vi "HFRR ADV v020 new software.vi"() -> ()   [LabVIEW 2025] (continued)
                  n3417 = local write "S 59"(w4556) -> ()
                }
                frame 59 {
                  n3418 = local write "S 60"(w4557) -> ()
                }
                frame 60 {
                  n3419 = local write "S 62"(w4558) -> ()
                }
                frame 61 {
                  n3420 = local write "S 63"(w4559) -> ()
                }
                frame 62 {
                  n3421 = local write "S 64"(w4560) -> ()
                }
                frame 63 {
                  n3422 = local write "S 65"(w4561) -> ()
                }
                frame 64 {
                  n3423 = local write "S 66"(w4562) -> ()
                }
                frame 65 {
                  n3424 = local write "S 67"(w4563) -> ()
                }
                frame 66 {
                  n3425 = local write "S 68"(w4564) -> ()
                }
                frame 67 {
                  n3426 = local write "S 69"(w4565) -> ()
                }
                frame 68 {
                  n3427 = local write "S 70"(w4566) -> ()
                }
                frame 69 {
                  n3428 = local write "S 71"(w4567) -> ()
                }
                frame 70 {
                  n3429 = local write "S 72"(w4568) -> ()
                }
                frame 71 {
                  n3430 = local write "S 73"(w4569) -> ()
                }
                frame 72 {
                  n3431 = local write "S 74"(w4570) -> ()
                }
                frame 73 {
                  n3432 = local write "S 75"(w4571) -> ()
                }
                frame 74 {
                  n3433 = local write "S 76"(w4572) -> ()
                }
                frame 75 {
                  n3434 = local write "S 77"(w4573) -> ()
                }
                frame 76 {
                  n3435 = local write "S 78"(w4574) -> ()
                }
                frame 77 {
                  n3436 = local write "S 79"(w4575) -> ()
                }
                frame 79 {
                  n3437 = property on="Sample Temperature ( °C )" class="XYGraph (strict)"("Y Scale.Name Label.Text"=w4576) -> ()  [unwired: 2 in, 2 out]
                }
                frame 80 {
                  n3438 = local write "S 81"(w4577) -> ()
                  n3439 = property on="Humidity ( %RH )" class="XYGraph (strict)"("Y Scale.Name Label.Text"=w4577) -> ()  [unwired: 2 in, 2 out]
                }
                frame 78 {
                  n3440 = property on="Air Temperature  ( °C )" class="XYGraph (strict)"("X Scale.Name Label.Text"=w4578) -> ()  [unwired: 2 in, 2 out]
                  n3441 = property on="Humidity ( %RH )" class="XYGraph (strict)"("X Scale.Name Label.Text"=w4578) -> ()  [unwired: 2 in, 2 out]
                  n3442 = property on="Sample Temperature ( °C )" class="XYGraph (strict)"("X Scale.Name Label.Text"=w4578) -> ()  [unwired: 2 in, 2 out]
                  n3443 = property on="Coefficient Of Friction" class="XYGraph (strict)"("X Scale.Name Label.Text"=w4578) -> ()  [unwired: 2 in, 2 out]
                }
                frame 81 {
                  n3444 = property on="Air Temperature  ( °C )" class="XYGraph (strict)"("Y Scale.Name Label.Text"=w4579) -> ()  [unwired: 2 in, 2 out]
                }
                frame 82 {
                  n3445 = local write "S 84"(w4580) -> ()
                }
                frame 83 {
                  n3446 = local write "S 85"(w4581) -> ()
                }
                frame 84 {
                  n3447 = local write "S 86"(w4582) -> ()
                }
                frame 85 {
                  n3448 = local write "S 87"(w4583) -> ()
                }
                frame 86 {
                  n3449 = local write "S 88"(w4584) -> ()
                }
                frame 87 {
                }
                frame 88 {
                  n3450 = local write "S 90"(w4586) -> ()
                }
                frame 89 {
                  n3451 = local write "S 91"(w4587) -> ()
                }
                frame 90 {
                  n3452 = local write "S 92"(w4588) -> ()
                }
                frame 91 {
                  n3453 = local write "S 93"(w4589) -> ()
                }
                frame 92 {
                  n3454 = local write "S 94"(w4590) -> ()
                }
                frame 93 {
                  n3455 = local write "S 95"(w4591) -> ()
                }
                frame 94 {
                  n3456 = local write "S 96"(w4592) -> ()
                }
                frame 95 {
                  n3457 = local write "S 97"(w4593) -> ()
                }
                frame 96 {
                  n3458 = local write "S 98"(w4594) -> ()
                }
                frame 97 {
                  n3459 = local write "S 99"(w4595) -> ()
                }
                frame 98 {
                  n3460 = local write "S 100"(w4596) -> ()
                }
                frame 99 {
                  n3461 = local write "S 101"(w4597) -> ()
                }
                frame 100 {
                  n3462 = local write "S 102"(w4598) -> ()
                }
                frame 101 {
                  n3463 = local write "S 103"(w4599) -> ()
                }
                frame 102 {
                  n3464 = local write "S 104"(w4600) -> ()
                }
                frame 103 {
                  n3465 = local write "S 105"(w4601) -> ()
                }
                frame 104 {
                  n3466 = local write "S 106"(w4602) -> ()
                }
                frame 105 {
                }
                frame 106 {
                  n3467 = property on="OK Button 17" class="Bool (strict)"("Boolean Text.Text"=w4603) -> ()  [unwired: 2 in, 2 out]
                }
                frame 107 {
                  n3468 = property on="OK Button 16" class="Bool (strict)"("Boolean Text.Text"=w4604) -> ()  [unwired: 2 in, 2 out]
                }
                frame 108 {
                  n3469 = property on="TITTLE" class="Str"("Caption.Text"=w4605) -> ()  [unwired: 2 in, 2 out]
                }
                frame 109 {
                  "String 30" <- w4606
                }
                frame 110 {
                  n3470 = property on="Test Date" class="Str"("Caption.Text"=w4607) -> ()  [unwired: 2 in, 2 out]
                  "String 31" <- w4607
                }
                frame 111 {
                  n3471 = property on="Sample ID" class="Str"("Caption.Text"=w4608) -> ()  [unwired: 2 in, 2 out]
                  "String 32" <- w4608
                }
                frame 112 {
                  n3472 = property on="Tested by" class="Str"("Caption.Text"=w4609) -> ()  [unwired: 2 in, 2 out]
                  "String 33" <- w4609
                }
                frame 113 {
                  n3473 = property on="System Configured Printers 2" class="Arr (strict)"("Caption.Text"=w4610) -> ()  [unwired: 2 in, 2 out]
                }
                frame 114 {
                  n3474 = property on="Selected Printer" class="Str"("Caption.Text"=w4611) -> ()  [unwired: 2 in, 2 out]
                }
                frame 115 {
                  n3475 = property on="Select Printer 3" class="DigNum (strict)"("Caption.Text"=w4612) -> ()  [unwired: 2 in, 2 out]
                }
                frame 116 {
                  n3476 = property on="Print" class="Bool (strict)"("Boolean Text.Text"=w4613) -> ()  [unwired: 2 in, 2 out]
                }
                frame 117 {
                  "String 41" <- w4614
                }
                frame 118 {
                  n3477 = property on="tested by" class="Str"("Caption.Text"=w4615) -> ()  [unwired: 2 in, 2 out]
                }
                frame 119 {
                }
                frame 120 {
                  n3478 = property on="Export" class="Bool (strict)"("Boolean Text.Text"=w4616) -> ()  [unwired: 2 in, 2 out]
                }
                frame 121 {
                  n3479 = property on="TEMP INTERCEPT:" class="DigNum (strict)"("Caption.Text"=w4617) -> ()  [unwired: 2 in, 2 out]
                }
                frame 122 {
                  n3480 = property on="AIR TEMP INTERCEPT:" class="DigNum (strict)"("Caption.Text"=w4618) -> ()  [unwired: 2 in, 2 out]
                }
                frame 123 {
                  n3481 = property on="Select File Type" class="Enum (strict)"("Caption.Text"=w4619) -> ()  [unwired: 2 in, 2 out]
                }
                frame 124 {
                  n3482 = property on="s.NO" class="Str"("Caption.Text"=w4620) -> ()  [unwired: 2 in, 2 out]
                  "String 45" <- w4620
                }
                frame 125 {
                  n3483 = property on="trip1 8" class="Bool (strict)"("Boolean Text.Text"=w4621) -> ()  [unwired: 2 in, 2 out]
                }
                frame 126, Default {
                }
              }
            }
          }
          frame #1 {
            w4629 = TRUE ("Visible")
            n3484 = local read "S 91"() -> (w4646:string)
            n3485 = local read "S 90"() -> (w4645:string)
            n3486 = local read "S 88"() -> (w4644:string)
            n3487 = property on="File Path" class="Path"("Caption.Text"=w4645) -> ()  [unwired: 2 in, 2 out]
            n3488 = property on="SrvM CP" class="Bool (strict)"("Boolean Text.Text"=w4644) -> ()  [unwired: 2 in, 2 out]
            n3489 = local read "S 71"() -> (w4639:string)
            n3490 = local read "S 86"() -> (w4641:string)
            n3491 = local read "S 85"() -> (w4642:string)
            n3492 = local read "S 87"() -> (w4640:string)
            n3493 = local read "S 84"() -> (w4643:string)
            n3494 = local read "S 103"() -> (w4628:string)
            n3495 = local read "S 104"() -> (w4627:string)
            n3496 = property on="ENTER THE NEW PASSWORD" class="Str"("Caption.Text"=w4640) -> ()  [unwired: 2 in, 2 out]
            n3497 = property on="Password" class="Str"("Caption.Text"=w4642) -> ()  [unwired: 2 in, 2 out]
            n3498 = property on="ENTER CURRENT PASSWORD" class="Str"("Caption.Text"=w4641) -> ()  [unwired: 2 in, 2 out]
            n3499 = property on="EDIT" class="Bool (strict)"("Boolean Text.Text"=w4639) -> ()  [unwired: 2 in, 2 out]
            n3500 = property on="SAVE" class="Bool (strict)"("Boolean Text.Text"=w4643) -> ()  [unwired: 2 in, 2 out]
            n3501 = Build Array(w4628, w4627) -> (w4626:string[])
            n3502 = property on="Heater Button" class="Bool (strict)"("Strings [4]"=w4626) -> ()  [unwired: 2 in, 2 out]
            n3503 = property on="CH-HUMIDITY WET" class="DigNum (strict)"("Caption.Size to Text?"=w4629) -> ()  [unwired: 2 in, 2 out]
            n3504 = property on="CH-HUMIDITY DRY" class="DigNum (strict)"("Caption.Size to Text?"=w4629) -> ()  [unwired: 2 in, 2 out]
            n3505 = property on="CH-POWER -" class="DigNum (strict)"("Caption.Size to Text?"=w4629) -> ()  [unwired: 2 in, 2 out]
            n3506 = property on="CH-HEATER" class="DigNum (strict)"("Caption.Size to Text?"=w4629) -> ()  [unwired: 2 in, 2 out]
            n3507 = property on="CH-POWER +" class="DigNum (strict)"("Caption.Size to Text?"=w4629) -> ()  [unwired: 2 in, 2 out]
            n3508 = local read "S 92"() -> (w4638:string)
            n3509 = local read "S 93"() -> (w4637:string)
            n3510 = local read "S 105"() -> (w4624:string)
            n3511 = local read "S 106"() -> (w4623:string)
            n3512 = Build Array(w4638, w4637) -> ()  [unwired: 1 out]
            n3513 = Build Array(w4624, w4623) -> (w4625:string[])
            n3514 = local read "S 95"() -> (w4635:string)
            n3515 = local read "S 94"() -> (w4636:string)
            n3516 = local read "bs"() -> (w4651:string)
            n3517 = local read "as"() -> (w4652:string)
            n3518 = property on="Humidity" class="Bool (strict)"("Strings [4]"=w4625) -> ()  [unwired: 2 in, 2 out]
            n3519 = Concatenate Strings(w4651, "\r", w4652) -> ()  [unwired: 1 out]
            n3520 = property on="STROKE GAIN :" class="DigNum (strict)"("Caption.Text"=w4635) -> ()  [unwired: 2 in, 2 out]
            n3521 = property on="DISPLACEMENT :" class="DigNum (strict)"("Caption.Text"=w4636) -> ()  [unwired: 2 in, 2 out]
            n3522 = property on="Rh After" class="DigNum (strict)"("Caption.Size to Text?"=TRUE ("Caption.Size to Text")) -> ()  [unwired: 2 in, 2 out]
            n3523 = local read "S 48"() -> (w4675:string)
            n3524 = local read "S 50"() -> (w4673:string)
            n3525 = local read "S 51"() -> (w4672:string)
            n3526 = local read "S 49"() -> (w4674:string)
            n3527 = local read "S 52"() -> (w4671:string)
            n3528 = local read "as"() -> (w4656:string)
            n3529 = local read "bs"() -> (w4657:string)
            n3530 = local read "S 56"() -> (w4670:string)
            n3531 = local read "S 57"() -> (w4669:string)
            n3532 = local read "S 58"() -> (w4668:string)
            n3533 = local read "S 59"() -> (w4667:string)
            n3534 = property on="OPEN" class="Bool (strict)"("Boolean Text.Text"=w4671) -> ()  [unwired: 2 in, 2 out]
            n3535 = property on="OPEN 1" class="Bool (strict)"("Boolean Text.Text"=w4675) -> ()  [unwired: 2 in, 2 out]
            n3536 = property on="OPEN 2" class="Bool (strict)"("Boolean Text.Text"=w4674) -> ()  [unwired: 2 in, 2 out]
            n3537 = property on="OPEN 3" class="Bool (strict)"("Boolean Text.Text"=w4673) -> ()  [unwired: 2 in, 2 out]
            n3538 = property on="OPEN 4" class="Bool (strict)"("Boolean Text.Text"=w4672) -> ()  [unwired: 2 in, 2 out]
            n3539 = Concatenate Strings(w4657, "\r", w4656) -> ()  [unwired: 1 out]
            n3540 = local read "S 102"() -> (w4630:string)
            n3541 = property on="КОФ1" class="DigNum (strict)"("Caption.Text"=w4670) -> ()  [unwired: 2 in, 2 out]
            n3542 = local read "S 98"() -> (w4634:string)
            n3543 = local read "S 99"() -> (w4633:string)
            n3544 = local read "S 100"() -> (w4632:string)
            n3545 = local read "S 101"() -> (w4631:string)
            n3546 = property on="КОФ2" class="DigNum (strict)"("Caption.Text"=w4669) -> ()  [unwired: 2 in, 2 out]
            n3547 = property on="КОФ3" class="DigNum (strict)"("Caption.Text"=w4668) -> ()  [unwired: 2 in, 2 out]
            n3548 = property on="КОФ4" class="DigNum (strict)"("Caption.Text"=w4667) -> ()  [unwired: 2 in, 2 out]
            n3549 = local read "bs"() -> (w4655:string)
            n3550 = local read "as"() -> (w4654:string)
            n3551 = property on="CH-POWER +" class="DigNum (strict)"("Caption.Text"=w4634) -> ()  [unwired: 2 in, 2 out]
            n3552 = property on="CH-POWER -" class="DigNum (strict)"("Caption.Text"=w4633) -> ()  [unwired: 2 in, 2 out]
            n3553 = property on="CH-HEATER" class="DigNum (strict)"("Caption.Text"=w4632) -> ()  [unwired: 2 in, 2 out]
            n3554 = property on="CH-HUMIDITY DRY" class="DigNum (strict)"("Caption.Text"=w4631) -> ()  [unwired: 2 in, 2 out]
            n3555 = property on="CH-HUMIDITY WET" class="DigNum (strict)"("Caption.Text"=w4630) -> ()  [unwired: 2 in, 2 out]
            n3556 = local read "S 60"() -> (w4666:string)
            n3557 = local read "S 54"() -> (w4676:string)
            n3558 = Concatenate Strings(w4655, "\r", w4654) -> ()  [unwired: 1 out]
            n3559 = Concatenate Strings(w4676, w4666) -> ()  [unwired: 1 out]
            n3560 = local read "S 77"() -> (→"String 43":string)
            n3561 = local read "S 76"() -> (w4649:string)
            n3562 = local read "S 78"() -> (w4648:string)
            n3563 = local read "S 71"() -> (w4660:string)
            n3564 = local read "S 66"() -> (w4665:string)
            n3565 = local read "S 67"() -> (w4664:string)
            n3566 = local read "S 68"() -> (w4663:string)
            n3567 = local read "S 69"() -> (w4662:string)
            n3568 = local read "S 70"() -> (w4661:string)
            n3569 = property on="AIR TEMP" class="DigNum (strict)"("Caption.Text"=w4648) -> ()  [unwired: 2 in, 2 out]
            n3570 = property on="Set Strk" class="DigNum (strict)"("Caption.Text"=w4649) -> ()  [unwired: 2 in, 2 out]
            n3571 = property on="FRIC. FORCE :" class="DigNum (strict)"("Caption.Text"=w4665) -> ()  [unwired: 2 in, 2 out]
            n3572 = property on="TEMPERATURE :" class="DigNum (strict)"("Caption.Text"=w4664) -> ()  [unwired: 2 in, 2 out]
            n3573 = property on="SPEED OUT:" class="DigNum (strict)"("Caption.Text"=w4663) -> ()  [unwired: 2 in, 2 out]
            n3574 = property on="AIR TEMPERATURE :" class="DigNum (strict)"("Caption.Text"=w4662) -> ()  [unwired: 2 in, 2 out]
            n3575 = property on="HUMIDITY:" class="DigNum (strict)"("Caption.Text"=w4661) -> ()  [unwired: 2 in, 2 out]
            n3576 = property on="EDIT" class="Bool (strict)"("Boolean Text.Text"=w4660) -> ()  [unwired: 2 in, 2 out]
            n3577 = local read "S 79"() -> (w4647:string)
          }
          frame #2 {
          }
        }
        n3578 = local write "Lan flag"(10.0 ("Lan flag")) -> ()
      }
      frame Enabled {
      }
    }
    n3579 = Wait (ms)(milliseconds to wait=u32 2000) -> ()  [unwired: 1 out]
    n3580 = local read "Quit"() -> (w4450:bool)
  }
  n3581 = while {
    shift-right: [w4682] -> _
    shift-left: _ -> [w4683]
    shift-right: [w4680] -> _
    shift-left: T18 {"Read Heave and Surge"="", "Bytes at Heave Port"=0.0, "Heave and Surge COM Port:"="COM9", "Com Port 2"="COM7", "Residual Due"="", "Heave COM Status 2"=TRUE, "Heave COM Status"=TRUE, "Port 2"=TRUE, "Sway PPR"=6400.0, "Surge PPR"=6400.0, "Heave PPR"=6400.0, "Sway Pitch"=2.0, "Surge Pitch"=3.0, "Heave Pitch"=4.0, "Sway Pulses/mm"=320.0, "Surge Pulses/mm"=1600.0, "Heave Pulses/mm"=1600.0, "inner loop"=0.0, "Read Heave and Surge 2"="", "String 36"="", "Write S"=FALSE, "WriteCC1"=[""], "Heave COM Loop"=0, "LastCom"="", "EXIT"=FALSE, "Error Heave"={"status"=TRUE, "code"=-1073807343, "source"=""}} -> [w4679]
    shift-right: [w4677] -> _
    shift-left: enum16{"init", "MAIN", "Panel Close"}."init" -> [w4678]
    stop <- w4681 stop-if-true
    n3582 = case shown="\"MAIN\"" w4678 {
      tunnel: w4683 -> [w4697 w4713 w4773 w4775]
      tunnel: [w4692 w4721 w4773 w4775] -> w4682
      tunnel: [_ _ TRUE _] -> w4681
      tunnel: [w4688 w4719 w4771 w4774] -> w4680
      tunnel: w4679 -> [w4694 w4712 w4771 w4774]
      tunnel: [enum16{"init", "MAIN", "Panel Close"}."MAIN" w4707 _ _] -> w4677
      frame "init" {
        n3583 = local read "Com Port 1"() -> (w4684:refnum<visa-resource-name>)
        n3584 = Bundle By Name(cluster=w4694, "Heave and Surge COM Port:"=w4684) -> (w4693:T18)
        n3585 = call "Instrument fgv uno.vi"("Enum"=T31."INIT", "error in (no error) 2"=w4697, "INPUT"=w4693) -> ("error"=w4695:errorcluster, "output"=w4691:T18)  [unwired: 6 in, 1 out]
        n3586 = case shown="Error" w4695 {
          selector: w4695 -> [w4699 _]
          tunnel: [w4699 w4703] -> w4692
          tunnel: w4691 -> [w4698 w4701]
          tunnel: [w4698 w4700] -> w4689
          frame No Error {
          }
          frame Error {
            n3587 = call "Instrument fgv uno.vi"("Enum"=T31."ERROR INIT", "INPUT"=w4701) -> ("error"=w4704:errorcluster, "output"=w4700:T18)  [unwired: 7 in, 1 out]
            n3588 = call <vilib>:"Clear Errors.vi"("error in (no error)"=w4704) -> ("error out"=w4703:errorcluster)  [unwired: 5 in, 1 out]
          }
        }
        n3589 = local read "LastCom 2"() -> (w4687:string)
        n3590 = Unbundle By Name(w4689) -> ("Heave COM Status 2"=→"COM Status 2" →"Instrument Status 2":bool, "Error Heave"=→"Error  2":errorcluster)  [unwired: 1 out]
        n3591 = Bundle By Name(cluster=w4689, "LastCom"=w4687) -> (w4688:T18)
      }
      frame "MAIN" {
        n3592 = Unbundle By Name(w4712) -> ("Com Port 2"=w4723:refnum<visa-resource-name>)
        n3593 = local read "Com Port 1"() -> (w4706:refnum<visa-resource-name>)
        n3594 = local write "Com Port 5"(w4723) -> ()
        n3595 = Bundle By Name(cluster=w4712, "Heave and Surge COM Port:"=w4706) -> (w4711:T18)
        n3596 = Equal?(x=w4723, y=w4706) -> (x = y?=w4722:bool)
        n3597 = case shown="True" w4722 {
          tunnel: [w4727 w4744] -> w4721
          tunnel: w4713 -> [w4728 w4750]
          tunnel: w4711 -> [w4726 w4748]
          tunnel: [w4725 w4743] -> w4719
          frame False {
            n3598 = call <vilib>:"Clear Errors.vi"("error in (no error)"=w4728) -> ("error out"=w4724:errorcluster)  [unwired: 5 in, 1 out]
            n3599 = call "Instrument fgv uno.vi"("Enum"=T31."ERROR INIT", "error in (no error) 2"=w4724, "INPUT"=w4726) -> ("error"=w4730:errorcluster, "output"=w4725:T18)  [unwired: 6 in, 1 out]
            n3600 = call <vilib>:"Clear Errors.vi"("error in (no error)"=w4730) -> ("error out"=w4727:errorcluster)  [unwired: 5 in, 1 out]
          }
          frame True {
            n3601 = call "Instrument fgv uno.vi"("Enum"=T31."READ", "error in (no error) 2"=w4750, "INPUT"=w4748) -> ("error"=w4749:errorcluster, "output"=w4740:T18)  [unwired: 6 in, 1 out]
            n3602 = Bundle By Name(cluster=w4740, "String 36"="String 15") -> (w4739:T18)
            n3603 = case shown="True" "Write S 2" {
              selector: "Write S 2" -> [_ w4770]
              tunnel: w4749 -> [w4763 w4769]
              tunnel: [w4763 w4768] -> w4736
              tunnel: w4739 -> [w4762 w4765]
              tunnel: [w4762 w4764] -> w4735
              frame False {
              }
              frame True {
                n3604 = Not(x=w4770) -> (.not. x?=w4766:bool)
                n3605 = local write "Write S 2"(w4766) -> ()
                n3606 = call "Instrument fgv uno.vi"("Enum"=T31."MANUAL WRITE", "error in (no error) 2"=w4769, "INPUT"=w4765) -> ("error"=w4768:errorcluster, "output"=w4764:T18)  [unwired: 6 in, 1 out]
              }
            }
            n3607 = Array Size(array="WriteHumidity") -> (size(s)=w4733:i32)
            n3608 = Greater Than 0?(x=w4733) -> (x > 0?=w4732:bool)
            n3609 = call "Instrument fgv uno.vi"("Enum"=T31."WRITE", "error in (no error) 2"=w4736, "WriteCC1"="WriteHumidity", "INPUT"=w4735) -> ("error"=w4746:errorcluster, "WriteCC1 2"=w4734:string[], "output"=w4745:T18)  [unwired: 5 in]
            n3610 = case shown="True" w4732 {
              tunnel: w4734 -> [_ w4752]
              frame False {
              }
              frame True {
                n3611 = local write "WriteHumidity 2"(w4752) -> ()
              }
            }
            n3612 = case shown="No Error" w4746 {
              selector: w4746 -> [w4753 w4756]
              tunnel: w4745 -> [w4754 w4761]
              tunnel: [w4754 w4760] -> w4743
              tunnel: [w4753 w4758] -> w4744
              frame No Error {
              }
              frame Error {
                n3613 = call <vilib>:"Clear Errors.vi"("error in (no error)"=w4756) -> ("error out"=w4755:errorcluster)  [unwired: 5 in, 1 out]
                n3614 = call "Instrument fgv uno.vi"("Enum"=T31."ERROR INIT", "error in (no error) 2"=w4755, "INPUT"=w4761) -> ("error"=w4759:errorcluster, "output"=w4760:T18)  [unwired: 6 in, 1 out]
                n3615 = call <vilib>:"Clear Errors.vi"("error in (no error)"=w4759) -> ("error out"=w4758:errorcluster)  [unwired: 5 in, 1 out]
              }
            }
            n3616 = Unbundle By Name(w4743) -> ("LastCom"=→"LastCom 2":string, "Read Heave and Surge"=→"Read Uno":string)
          }
        }
        n3617 = Unbundle By Name(w4719) -> ("Heave COM Status 2"=w4720:bool, "Heave COM Status"=w4705:bool, "Error Heave"=w4717:errorcluster, "Bytes at Heave Port"=→"Bytes at Humidity Port  2":dbl)
        n3618 = Unbundle By Name(w4717) -> ("status"=→"Humidity Port 2":bool)
        n3619 = Not(x=w4705) -> (.not. x?=w4714:bool)
        n3620 = local write "Error  2"(w4717) -> ()
        n3621 = Not(x=w4720) -> (.not. x?=w4715:bool)
        n3622 = local write "Instrument Status 2"(w4714) -> ()
        n3623 = local write "COM Status 2"(w4715) -> ()
        n3624 = local write "Port 1a"(w4705) -> ()
        n3625 = local read "Quit"() -> (w4708:bool)
        n3626 = Select(t=enum16{"init", "MAIN", "Panel Close"}."Panel Close", s=w4708, f=enum16{"init", "MAIN", "Panel Close"}."MAIN") -> (s? t:f=w4707:enum16{"init", "MAIN", "Panel Close"})
      }
      frame "Panel Close" {
      }
      frame Default {
      }
    }
  }
  n3627 = disable-structure shown="Disabled" {
    frame Disabled {
      n3628 = while {
        tunnel: [w4777] -> _
        i -> [w4777]
        stop <- w4776 continue-if-true
        n3629 = Wait (ms)(milliseconds to wait=u32 50) -> ()  [unwired: 1 out]
        n3630 = stacked-sequence {
          frame #0 {
            # "Controls Text color"
            # "Controls BG color"
            n3631 = property on="FILE" class="Str"("Text.Text Colors:Text Color"="SC  Text") -> ()  [unwired: 2 in, 2 out]
            n3632 = property on="Fuel Discription :" class="Str"("Text.Text Colors:Text Color"="SC  Text") -> ()  [unwired: 2 in, 2 out]
            n3633 = property on="tested by" class="Str"("Text.Text Colors:Text Color"="SC  Text") -> ()  [unwired: 2 in, 2 out]
            n3634 = property on="Remarks :" class="Str"("Text.Text Colors:Text Color"="SC  Text") -> ()  [unwired: 2 in, 2 out]
            n3635 = property class="DigNum (strict)"("Numeric Text.Text Colors:BG Color"="NC BG") -> ()  [unwired: 2 in, 2 out]
            n3636 = property class="DigNum (strict)"("Numeric Text.Text Colors:BG Color"="NC BG") -> ()  [unwired: 2 in, 2 out]
            n3637 = property class="DigNum (strict)"("Numeric Text.Text Colors:BG Color"="NC BG") -> ()  [unwired: 2 in, 2 out]
            n3638 = property class="DigNum (strict)"("Numeric Text.Text Colors:BG Color"="NC BG") -> ()  [unwired: 2 in, 2 out]
            n3639 = property class="DigNum (strict)"("Numeric Text.Text Colors:BG Color"="NC BG") -> ()  [unwired: 2 in, 2 out]
            n3640 = property class="DigNum (strict)"("Numeric Text.Text Colors:BG Color"="NC BG") -> ()  [unwired: 2 in, 2 out]
            n3641 = property class="DigNum (strict)"("Numeric Text.Text Colors:BG Color"="NC BG") -> ()  [unwired: 2 in, 2 out]
            n3642 = property class="DigNum (strict)"("Numeric Text.Text Colors:BG Color"="NC BG") -> ()  [unwired: 2 in, 2 out]
            n3643 = property class="DigNum (strict)"("Numeric Text.Text Colors:BG Color"="NC BG") -> ()  [unwired: 2 in, 2 out]
            n3644 = property class="DigNum (strict)"("Numeric Text.Text Colors:BG Color"="NC BG") -> ()  [unwired: 2 in, 2 out]
            n3645 = property class="DigNum (strict)"("Numeric Text.Text Colors:BG Color"="NC BG") -> ()  [unwired: 2 in, 2 out]
            n3646 = property class="DigNum (strict)"("Numeric Text.Text Colors:BG Color"="NC BG") -> ()  [unwired: 2 in, 2 out]
            n3647 = property on="FILE" class="Str"("Text.Text Colors:BG Color"="SC BG 3") -> ()  [unwired: 2 in, 2 out]
            n3648 = property on="Fuel Discription :" class="Str"("Text.Text Colors:BG Color"="SC BG 3") -> ()  [unwired: 2 in, 2 out]
            n3649 = property on="tested by" class="Str"("Text.Text Colors:BG Color"="SC BG 3") -> ()  [unwired: 2 in, 2 out]
            n3650 = property on="Remarks :" class="Str"("Text.Text Colors:BG Color"="SC BG 3") -> ()  [unwired: 2 in, 2 out]
            n3651 = property class="DigNum (strict)"("Numeric Text.Text Colors:Text Color"="NC Text") -> ()  [unwired: 2 in, 2 out]
            n3652 = property class="DigNum (strict)"("Numeric Text.Text Colors:Text Color"="NC Text") -> ()  [unwired: 2 in, 2 out]
            n3653 = property class="DigNum (strict)"("Numeric Text.Text Colors:Text Color"="NC Text") -> ()  [unwired: 2 in, 2 out]
            n3654 = property class="DigNum (strict)"("Numeric Text.Text Colors:Text Color"="NC Text") -> ()  [unwired: 2 in, 2 out]
            n3655 = property class="DigNum (strict)"("Numeric Text.Text Colors:Text Color"="NC Text") -> ()  [unwired: 2 in, 2 out]
            n3656 = property class="DigNum (strict)"("Numeric Text.Text Colors:Text Color"="NC Text") -> ()  [unwired: 2 in, 2 out]
            n3657 = property class="DigNum (strict)"("Numeric Text.Text Colors:Text Color"="NC Text") -> ()  [unwired: 2 in, 2 out]
            n3658 = property class="DigNum (strict)"("Numeric Text.Text Colors:Text Color"="NC Text") -> ()  [unwired: 2 in, 2 out]
            n3659 = property class="DigNum (strict)"("Numeric Text.Text Colors:Text Color"="NC Text") -> ()  [unwired: 2 in, 2 out]
            n3660 = property class="DigNum (strict)"("Numeric Text.Text Colors:Text Color"="NC Text") -> ()  [unwired: 2 in, 2 out]
            n3661 = property class="DigNum (strict)"("Numeric Text.Text Colors:Text Color"="NC Text") -> ()  [unwired: 2 in, 2 out]
            n3662 = property class="DigNum (strict)"("Numeric Text.Text Colors:Text Color"="NC Text") -> ()  [unwired: 2 in, 2 out]
            n3663 = property class="DigNum (strict)"("Numeric Text.Text Colors:Text Color"="NI Text  2") -> ()  [unwired: 2 in, 2 out]
            n3664 = property class="DigNum (strict)"("Numeric Text.Text Colors:Text Color"="NI Text  2") -> ()  [unwired: 2 in, 2 out]
            n3665 = property class="DigNum (strict)"("Numeric Text.Text Colors:Text Color"="NI Text  2") -> ()  [unwired: 2 in, 2 out]
            n3666 = property class="DigNum (strict)"("Numeric Text.Text Colors:Text Color"="NI Text  2") -> ()  [unwired: 2 in, 2 out]
            n3667 = property class="DigNum (strict)"("Numeric Text.Text Colors:Text Color"="NI Text  2") -> ()  [unwired: 2 in, 2 out]
            n3668 = property class="DigNum (strict)"("Numeric Text.Text Colors:Text Color"="NI Text  2") -> ()  [unwired: 2 in, 2 out]
            n3669 = property class="DigNum (strict)"("Numeric Text.Text Colors:Text Color"="NI Text  2") -> ()  [unwired: 2 in, 2 out]
            n3670 = property class="DigNum (strict)"("Numeric Text.Text Colors:Text Color"="NI Text  2") -> ()  [unwired: 2 in, 2 out]
            n3671 = property class="DigNum (strict)"("Numeric Text.Text Colors:Text Color"="NI Text  2") -> ()  [unwired: 2 in, 2 out]
            n3672 = property class="DigNum (strict)"("Numeric Text.Text Colors:Text Color"="NI Text  2") -> ()  [unwired: 2 in, 2 out]
            n3673 = property class="DigNum (strict)"("Numeric Text.Text Colors:Text Color"="NI Text  2") -> ()  [unwired: 2 in, 2 out]
            n3674 = property class="DigNum (strict)"("Numeric Text.Text Colors:Text Color"="NI Text  2") -> ()  [unwired: 2 in, 2 out]
            n3675 = property class="DigNum (strict)"("Numeric Text.Text Colors:Text Color"="NI Text  2") -> ()  [unwired: 2 in, 2 out]
            n3676 = property class="DigNum (strict)"("Numeric Text.Text Colors:Text Color"="NI Text  2") -> ()  [unwired: 2 in, 2 out]
            n3677 = property class="DigNum (strict)"("Numeric Text.Text Colors:Text Color"="NI Text  2") -> ()  [unwired: 2 in, 2 out]
            n3678 = property on="Coefficient Of Friction" class="XYGraph (strict)"("Plot Area:Colors:FG Color"="GFG  2", "Plot Area:Colors:BG Color"="GBG   2") -> ()  [unwired: 2 in, 2 out]
            n3679 = property on="Humidity ( %RH )" class="XYGraph (strict)"("Plot Area:Colors:FG Color"="GFG  2", "Plot Area:Colors:BG Color"="GBG   2") -> ()  [unwired: 2 in, 2 out]
            n3680 = property on="Air Temperature  ( °C )" class="XYGraph (strict)"("Plot Area:Colors:FG Color"="GFG  2", "Plot Area:Colors:BG Color"="GBG   2") -> ()  [unwired: 2 in, 2 out]
            n3681 = property on="Sample Temperature ( °C )" class="XYGraph (strict)"("Plot Area:Colors:FG Color"="GFG  2", "Plot Area:Colors:BG Color"="GBG   2") -> ()  [unwired: 2 in, 2 out]
            n3682 = property class="DigNum (strict)"("Numeric Text.Text Colors:BG Color"="NI BG 2") -> ()  [unwired: 2 in, 2 out]
            n3683 = property class="DigNum (strict)"("Numeric Text.Text Colors:BG Color"="NI BG 2") -> ()  [unwired: 2 in, 2 out]
            n3684 = property class="DigNum (strict)"("Numeric Text.Text Colors:BG Color"="NI BG 2") -> ()  [unwired: 2 in, 2 out]
            n3685 = property class="DigNum (strict)"("Numeric Text.Text Colors:BG Color"="NI BG 2") -> ()  [unwired: 2 in, 2 out]
            n3686 = property class="DigNum (strict)"("Numeric Text.Text Colors:BG Color"="NI BG 2") -> ()  [unwired: 2 in, 2 out]
            n3687 = property class="DigNum (strict)"("Numeric Text.Text Colors:BG Color"="NI BG 2") -> ()  [unwired: 2 in, 2 out]
            n3688 = property class="DigNum (strict)"("Numeric Text.Text Colors:BG Color"="NI BG 2") -> ()  [unwired: 2 in, 2 out]
            n3689 = property class="DigNum (strict)"("Numeric Text.Text Colors:BG Color"="NI BG 2") -> ()  [unwired: 2 in, 2 out]
            n3690 = property class="DigNum (strict)"("Numeric Text.Text Colors:BG Color"="NI BG 2") -> ()  [unwired: 2 in, 2 out]
            n3691 = property class="DigNum (strict)"("Numeric Text.Text Colors:BG Color"="NI BG 2") -> ()  [unwired: 2 in, 2 out]
            n3692 = property class="DigNum (strict)"("Numeric Text.Text Colors:BG Color"="NI BG 2") -> ()  [unwired: 2 in, 2 out]
            n3693 = property class="DigNum (strict)"("Numeric Text.Text Colors:BG Color"="NI BG 2") -> ()  [unwired: 2 in, 2 out]
            n3694 = property class="DigNum (strict)"("Numeric Text.Text Colors:BG Color"="NI BG 2") -> ()  [unwired: 2 in, 2 out]
            n3695 = property class="DigNum (strict)"("Numeric Text.Text Colors:BG Color"="NI BG 2") -> ()  [unwired: 2 in, 2 out]
            n3696 = property class="DigNum (strict)"("Numeric Text.Text Colors:BG Color"="NI BG 2") -> ()  [unwired: 2 in, 2 out]
            n3697 = property class="Bool"("Colors [4]"="Boolean BC T & BG") -> ()  [unwired: 2 in, 2 out]
            n3698 = property on="Save & Continue" class="Bool (strict)"("Colors [4]"="Boolean BC T & BG") -> ()  [unwired: 2 in, 2 out]
            n3699 = property on="Heater Button" class="Bool (strict)"("Colors [4]"="Boolean BC T & BG") -> ()  [unwired: 2 in, 2 out]
            n3700 = property class="Bool"("Colors [4]"="Boolean BC T & BG") -> ()  [unwired: 2 in, 2 out]
            n3701 = property on="Humidity" class="Bool (strict)"("Colors [4]"="Boolean BC T & BG") -> ()  [unwired: 2 in, 2 out]
            n3702 = property class="Bool (strict)"("Colors [4]"="Boolean BC T & BG") -> ()  [unwired: 2 in, 2 out]
            n3703 = property on="RUN" class="Bool (strict)"("Colors [4]"="Boolean BC T & BG") -> ()  [unwired: 2 in, 2 out]
            n3704 = property on="trip1 8" class="Bool (strict)"("Colors [4]"="Boolean BC T & BG") -> ()  [unwired: 2 in, 2 out]
            n3705 = property class="Bool"("Colors [4]"="Boolean BC T & BG") -> ()  [unwired: 2 in, 2 out]
            n3706 = property class="Bool (strict)"("Colors [4]"="Boolean BC T & BG") -> ()  [unwired: 2 in, 2 out]
            n3707 = property on="OPEN 1" class="Bool (strict)"("Colors [4]"="Boolean BC T & BG 2") -> ()  [unwired: 2 in, 2 out]
            n3708 = property on="OPEN 2" class="Bool (strict)"("Colors [4]"="Boolean BC T & BG 2") -> ()  [unwired: 2 in, 2 out]
            n3709 = property on="OPEN 3" class="Bool (strict)"("Colors [4]"="Boolean BC T & BG 2") -> ()  [unwired: 2 in, 2 out]
            n3710 = property on="OPEN 4" class="Bool (strict)"("Colors [4]"="Boolean BC T & BG 2") -> ()  [unwired: 2 in, 2 out]
            n3711 = property on="OPEN" class="Bool (strict)"("Colors [4]"="Boolean BC T & BG 2") -> ()  [unwired: 2 in, 2 out]
            n3712 = property on="rstv2" class="Bool"("Colors [4]"="Boolean BC T & BG 2") -> ()  [unwired: 2 in, 2 out]
            n3713 = property on="RST CP" class="Bool"("Colors [4]"="Boolean BC T & BG 2") -> ()  [unwired: 2 in, 2 out]
            n3714 = property on="RSTV1 3" class="Bool"("Colors [4]"="Boolean BC T & BG 2") -> ()  [unwired: 2 in, 2 out]
            n3715 = property on="RSTV1 2" class="Bool"("Colors [4]"="Boolean BC T & BG 2") -> ()  [unwired: 2 in, 2 out]
          }
          frame #1 {
          }
        }
        n3716 = local read "Quit"() -> (w4776:bool)
      }
    }
    frame Enabled {
    }
  }
  n3717 = while {
    shift-right: [w4794] -> _
    shift-left: _ -> [w4795]
    shift-right: [w4792] -> _
    shift-left: T18 {"Read Heave and Surge"="", "Bytes at Heave Port"=0.0, "Heave and Surge COM Port:"="COM9", "Com Port 2"="COM7", "Residual Due"="", "Heave COM Status 2"=TRUE, "Heave COM Status"=TRUE, "Port 2"=TRUE, "Sway PPR"=6400.0, "Surge PPR"=6400.0, "Heave PPR"=6400.0, "Sway Pitch"=2.0, "Surge Pitch"=3.0, "Heave Pitch"=4.0, "Sway Pulses/mm"=320.0, "Surge Pulses/mm"=1600.0, "Heave Pulses/mm"=1600.0, "inner loop"=0.0, "Read Heave and Surge 2"="", "String 36"="", "Write S"=FALSE, "WriteCC1"=[""], "Heave COM Loop"=0, "LastCom"="", "EXIT"=FALSE, "Error Heave"={"status"=TRUE, "code"=-1073807343, "source"=""}} -> [w4791]
    shift-right: [w4789] -> _
    shift-left: enum16{"init", "MAIN", "Panel Close"}."init" -> [w4790]
    stop <- w4793 stop-if-true
    n3718 = case shown="\"MAIN\"" w4790 {
      tunnel: w4795 -> [w4809 w4824 w4885 w4887]
      tunnel: [w4803 w4833 w4885 w4887] -> w4794
      tunnel: [_ _ TRUE _] -> w4793
      tunnel: [w4799 w4830 w4883 w4886] -> w4792
      tunnel: w4791 -> [w4806 w4823 w4883 w4886]
      tunnel: [enum16{"init", "MAIN", "Panel Close"}."MAIN" w4817 _ _] -> w4789
      frame "init" {
        n3719 = Bundle By Name(cluster=w4806, "Heave and Surge COM Port:"="C3 :") -> (w4805:T18)
        n3720 = call "Instrument fgv.vi"("Enum"=T31."INIT", "error in (no error) 2"=w4809, "INPUT"=w4805) -> ("error"=w4807:errorcluster, "output"=w4802:T18)  [unwired: 6 in, 1 out]
        n3721 = case shown="Error" w4807 {
          selector: w4807 -> [w4811 _]
          tunnel: [w4811 w4815] -> w4803
          tunnel: w4802 -> [w4810 w4813]
          tunnel: [w4810 w4812] -> w4800
          frame No Error {
          }
          frame Error {
            n3722 = call "Instrument fgv.vi"("Enum"=T31."ERROR INIT", "INPUT"=w4813) -> ("error"=w4816:errorcluster, "output"=w4812:T18)  [unwired: 7 in, 1 out]
            n3723 = call <vilib>:"Clear Errors.vi"("error in (no error)"=w4816) -> ("error out"=w4815:errorcluster)  [unwired: 5 in, 1 out]
          }
        }
        n3724 = local read "LastCom"() -> (w4798:string)
        n3725 = Unbundle By Name(w4800) -> ("Heave COM Status 2"=→"COM Status" →"Instrument Status":bool, "Error Heave"=→"Error":errorcluster)  [unwired: 1 out]
        n3726 = Bundle By Name(cluster=w4800, "LastCom"=w4798) -> (w4799:T18)
      }
      frame "MAIN" {
        n3727 = Unbundle By Name(w4823) -> ("Com Port 2"=w4835:refnum<visa-resource-name>)
        n3728 = local write "Com Port 4"(w4835) -> ()
        n3729 = local read "C3 :"() -> (w4821:refnum<visa-resource-name>)
        n3730 = Bundle By Name(cluster=w4823, "Heave and Surge COM Port:"=w4821) -> (w4822:T18)
        n3731 = Equal?(x=w4835, y=w4821) -> (x = y?=w4834:bool)
        n3732 = case shown="True" w4834 {
          tunnel: [w4839 w4856] -> w4833
          tunnel: w4824 -> [w4840 w4862]
          tunnel: w4822 -> [w4838 w4860]
          tunnel: [w4837 w4855] -> w4830
          frame False {
            n3733 = call <vilib>:"Clear Errors.vi"("error in (no error)"=w4840) -> ("error out"=w4836:errorcluster)  [unwired: 5 in, 1 out]
            n3734 = call "Instrument fgv.vi"("Enum"=T31."ERROR INIT", "error in (no error) 2"=w4836, "INPUT"=w4838) -> ("error"=w4842:errorcluster, "output"=w4837:T18)  [unwired: 6 in, 1 out]
            n3735 = call <vilib>:"Clear Errors.vi"("error in (no error)"=w4842) -> ("error out"=w4839:errorcluster)  [unwired: 5 in, 1 out]
          }
          frame True {
            n3736 = call "Instrument fgv.vi"("Enum"=T31."READ", "error in (no error) 2"=w4862, "INPUT"=w4860) -> ("error"=w4861:errorcluster, "output"=w4852:T18)  [unwired: 6 in, 1 out]
            n3737 = Bundle By Name(cluster=w4852, "String 36"="String 11") -> (w4851:T18)
            n3738 = case shown="True" "Write S" {
              selector: "Write S" -> [_ w4882]
              tunnel: w4861 -> [w4875 w4881]
              tunnel: [w4875 w4880] -> w4848
              tunnel: w4851 -> [w4874 w4877]
              tunnel: [w4874 w4876] -> w4847
              frame False {
              }
              frame True {
                n3739 = Not(x=w4882) -> (.not. x?=w4878:bool)
                n3740 = local write "Write S"(w4878) -> ()
                n3741 = call "Instrument fgv.vi"("Enum"=T31."MANUAL WRITE", "error in (no error) 2"=w4881, "INPUT"=w4877) -> ("error"=w4880:errorcluster, "output"=w4876:T18)  [unwired: 6 in, 1 out]
              }
            }
            n3742 = Array Size(array="WriteHumidity 2") -> (size(s)=w4845:i32)
            n3743 = Greater Than 0?(x=w4845) -> (x > 0?=w4844:bool)
            n3744 = call "Instrument fgv.vi"("Enum"=T31."WRITE", "error in (no error) 2"=w4848, "WriteCC1"="WriteHumidity 2", "INPUT"=w4847) -> ("error"=w4858:errorcluster, "WriteCC1 2"=w4846:string[], "output"=w4857:T18)  [unwired: 5 in]
            n3745 = case shown="True" w4844 {
              tunnel: w4846 -> [_ w4864]
              frame False {
              }
              frame True {
                n3746 = local write "WriteHumidity 2"(w4864) -> ()
              }
            }
            n3747 = case shown="Error" w4858 {
              selector: w4858 -> [w4865 w4868]
              tunnel: w4857 -> [w4866 w4873]
              tunnel: [w4866 w4872] -> w4855
              tunnel: [w4865 w4870] -> w4856
              frame No Error {
              }
              frame Error {
                n3748 = call <vilib>:"Clear Errors.vi"("error in (no error)"=w4868) -> ("error out"=w4867:errorcluster)  [unwired: 5 in, 1 out]
                n3749 = call "Instrument fgv.vi"("Enum"=T31."ERROR INIT", "error in (no error) 2"=w4867, "INPUT"=w4873) -> ("error"=w4871:errorcluster, "output"=w4872:T18)  [unwired: 6 in, 1 out]
                n3750 = call <vilib>:"Clear Errors.vi"("error in (no error)"=w4871) -> ("error out"=w4870:errorcluster)  [unwired: 5 in, 1 out]
              }
            }
            n3751 = Unbundle By Name(w4855) -> ("LastCom"=→"LastCom":string, "Read Heave and Surge"=→"Read Humidity":string)
          }
        }
        n3752 = Unbundle By Name(w4830) -> ("Heave COM Status 2"=w4832:bool, "Heave COM Status"=w4831:bool, "Error Heave"=w4828:errorcluster, "Bytes at Heave Port"=→"Bytes at Humidity Port":dbl)
        n3753 = Unbundle By Name(w4828) -> ("status"=→"Humidity Port":bool)
        n3754 = Not(x=w4831) -> (.not. x?=w4825:bool)
        n3755 = local write "Error"(w4828) -> ()
        n3756 = Not(x=w4832) -> (.not. x?=w4826:bool)
        n3757 = local write "Instrument Status"(w4825) -> ()
        n3758 = local write "COM Status"(w4826) -> ()
        n3759 = local read "Quit"() -> (w4818:bool)
        n3760 = Select(t=enum16{"init", "MAIN", "Panel Close"}."Panel Close", s=w4818, f=enum16{"init", "MAIN", "Panel Close"}."MAIN") -> (s? t:f=w4817:enum16{"init", "MAIN", "Panel Close"})
      }
      frame "Panel Close" {
      }
      frame Default {
      }
    }
  }
  n3761 = while {
    stop <- w4913 stop-if-true
    n3762 = local read "Read Uno"() -> (w4888:string)
    n3763 = call <vilib>:"High Resolution Polling Wait.vi"("seconds to wait"=0.05) -> ()  [unwired: 10 in, 1 out]
    n3764 = Spreadsheet String To Array(delimiter (Tab)=",", format string="", spreadsheet string=w4888, array type (2D Dbl)=string[] []) -> (array=w4908:string[])
    n3765 = for {
      tunnel: w4908 -> [w4918] mode=indexing
      tunnel: string[] ["STATE;", "SET;", "RH;", "T;", "AMB_RH;", "AMB_T;", "PUMP;", "FAN_IN;", "FAN_OUT;", "DEHUM;", "CURRENT;", "STALL;"] -> [w4917] mode=indexing
      tunnel: [w4916] -> w4907 mode=indexing
      n3766 = Match Pattern(string=w4918, regular expression=w4917) -> (after substring=w4916:string)  [unwired: 1 in, 3 out]
    }
    n3767 = Index Array(array=w4907) -> (element #1=→"STATE :":string, element #2=→"SET :":string, element #3=w4896:string, element #4=→"T :":string, element #5=w4894:string, element #6=→"AMB_T :":string, element #7=→"PUMP :":string, element #8=→"FAN_IN :":string, element #9=→"FAN_OUT :":string, element #10=→"DEHUM :":string, element #11=→"CURRENT :":string, element #12=→"STALL :":string)  [unwired: 12 in]
    "RH :" <- w4896
    "AMB_RH :" <- w4894
    n3768 = Fract/Exp String To Number(string=w4896) -> (number=w4889:dbl)  [unwired: 3 in, 1 out]
    n3769 = Fract/Exp String To Number(string=w4894) -> (number=w4893:dbl)  [unwired: 3 in, 1 out]
    n3770 = local write "Ambient Humidity :"(w4893) -> ()
    n3771 = Equal?(x=w4889, y=0.0) -> (x = y?=w4891:bool)
    n3772 = case shown="True" w4891 {
      tunnel: [w4914 w4915] -> w4890
      tunnel: w4889 -> [w4914 _]
      frame False {
        (unwired) 0.0
        "Humidity temp" <- w4914
      }
      frame True {
        n3773 = local read "Humidity temp"() -> (w4915:dbl)
      }
    }
    "RH Numeric:" <- w4890
    n3774 = local read "Quit"() -> (w4913:bool)
  }
  n3775 = disable-structure shown="Disabled" {
    frame Disabled {
      n3776 = while {
        tunnel: [w5152] -> _
        i -> [w5152]
        stop <- w5149 stop-if-true
        n3777 = local read "powstat"() -> (w5150:bool)
        n3778 = case shown="True" w5150 {
          frame False {
          }
          frame True {
            n3779 = local read "RUN"() -> (w5153:bool)
            n3780 = case shown="True" w5153 {
              frame False {
                w5183 = 65.0 ("y")
                n3781 = local read "Set Hz"() -> (w5211:dbl)
                n3782 = local read "NORMAL LOAD"() -> (w5212:dbl)
                n3783 = Multiply(x=w5211, y=60.0) -> (x*y=w5218:dbl)
                n3784 = Multiply(x=1.2 ("y"), y=0.949) -> (x*y=w5187:dbl)
                n3785 = Multiply(x=1.2 ("y"), y=0.8166) -> (x*y=w5191:dbl)
                n3786 = Multiply(x=1.2 ("y"), y=0.851) -> (x*y=w5186:dbl)
                n3787 = local read "FF 2"() -> (w5210:dbl)
                n3788 = Absolute Value(x=w5218) -> (abs(x)=w5216:dbl)
                n3789 = case shown="13.." w5210 {
                  tunnel: [1 2 3] -> w5208
                  frame 0..10, Default {
                    # "Normal"
                  }
                  frame 11, 12 {
                  }
                  frame 13.. {
                  }
                }
                "FF STATE" <- w5208
                n3790 = local read "TEMP"() -> (w5171:dbl)
                n3791 = local read item#-1() -> (w5185)
                n3792 = Less?(x=w5185, y=w5191) -> (x < y?=w5188:bool)
                n3793 = In Range and Coerce(upper limit=w5187, x=w5185, lower limit=w5186) -> (In Range?=w5189:bool)  [unwired: 1 out]
                n3794 = case shown="3601.." w5216 {
                  tunnel: [1 2 3] -> w5214
                  frame 0..3000, Default {
                    # "Normal"
                  }
                  frame 3001..3600 {
                  }
                  frame 3601.. {
                  }
                }
                n3795 = case shown="11.." w5212 {
                  tunnel: [1 3] -> w5213
                  frame 1..10, Default {
                  }
                  frame 11.. {
                  }
                }
                "NL STATE" <- w5213
                n3796 = Multiply(x=1.2 ("y"), y=0.95) -> (x*y=w5201:dbl)
                n3797 = Multiply(x=w5183, y=0.954) -> (x*y=w5175:dbl)
                n3798 = Or(x=w5188, y=w5189) -> (x .or. y?=w5190:bool)
                n3799 = Greater Or Equal?(x=w5185, y=w5201) -> (x >= y?=w5198:bool)
                n3800 = Multiply(x=w5183, y=0.99) -> (x*y=w5172:dbl)
                n3801 = Greater Or Equal?(x=w5171, y=w5172) -> (x >= y?=w5177:bool)
                n3802 = Greater Or Equal?(x=w5171, y=w5175) -> (x >= y?=w5174:bool)
                n3803 = case shown="0, 1, Default" w5185 {
                  tunnel: [1 3] -> w5202
                  frame 0, 1, Default {
                  }
                  frame 2.. {
                  }
                }
                n3804 = case shown="True" w5198 {
                  tunnel: [1 3] -> w5203
                  frame False {
                  }
                  frame True {
                  }
                }
                n3805 = case shown="True" w5190 {
                  tunnel: [1 2] -> w5204
                  frame False {
                  }
                  frame True {
                  }
                }
                n3806 = case shown="..0" w5171 {
                  tunnel: [2 3 3 1] -> w5178
                  frame 61, 62 {
                  }
                  frame 63.. {
                  }
                  frame ..0 {
                  }
                  frame 10..60, Default {
                  }
                }
                n3807 = case shown="True" w5177 {
                  tunnel: [1 3] -> w5179
                  frame False {
                  }
                  frame True {
                  }
                }
                n3808 = Number To Decimal String(number=w5214) -> (decimal integer string=w5215:string)  [unwired: 1 in]
                n3809 = case shown="True" w5174 {
                  tunnel: [1 2] -> w5180
                  frame False {
                  }
                  frame True {
                  }
                }
                n3810 = Number To Decimal String(number=1) -> (decimal integer string=→"Air temp":string)  [unwired: 1 in]
                n3811 = Number To Decimal String(number=w5208) -> (decimal integer string=→"ff_st":string)  [unwired: 1 in]
                n3812 = local write "sp_st"(w5215) -> ()
                n3813 = Number To Decimal String(number=w5213) -> (decimal integer string=→"nl_st":string)  [unwired: 1 in]
                n3814 = Build Array(w5178, w5179, w5180) -> (w5181:i32[])
                n3815 = Build Array(w5202, w5203, w5204) -> (w5205:i32[])
                n3816 = Array Max & Min(array=w5181) -> (max value=w5182:i32)  [unwired: 3 out]
                n3817 = Array Max & Min(array=w5205) -> (max value=w5206:i32)  [unwired: 3 out]
                n3818 = Number To Decimal String(number=w5182) -> (decimal integer string=w5170:string)  [unwired: 1 in]
                n3819 = Number To Decimal String(number=w5206) -> (decimal integer string=→"Stroke Ln 2":string)  [unwired: 1 in]
                n3820 = local write "temp_st"(w5170) -> ()
              }
              frame True {
                w5268 = 65.0 ("y")
                # "Healthy -1\nWarning -2\nError -3"
                n3821 = local read "TEMP"() -> (w5279:dbl)
                n3822 = local read "NORMAL LOAD"() -> (w5283:dbl)
                n3823 = local read "Set Hz"() -> (w5281:dbl)
                n3824 = Multiply(x=1.2 ("y"), y=0.949) -> (x*y=w5263:dbl)
                n3825 = Multiply(x=1.2 ("y"), y=0.8166) -> (x*y=w5259:dbl)
                n3826 = Multiply(x=1.2 ("y"), y=0.851) -> (x*y=w5264:dbl)
                n3827 = Multiply(x=w5268, y=0.954) -> (x*y=w5275:dbl)
                n3828 = Multiply(x=w5268, y=0.99) -> (x*y=w5278:dbl)
                n3829 = Greater Or Equal?(x=w5279, y=w5278) -> (x >= y?=w5273:bool)
                n3830 = Multiply(x=w5281, y=60.0) -> (x*y=w5287:dbl)
                n3831 = Greater Or Equal?(x=w5279, y=w5275) -> (x >= y?=w5276:bool)
                n3832 = local read "FF 2"() -> (w5282:dbl)
                n3833 = local read item#-1() -> (w5265)
                n3834 = Less?(x=w5265, y=w5259) -> (x < y?=w5262:bool)
                n3835 = In Range and Coerce(upper limit=w5263, x=w5265, lower limit=w5264) -> (In Range?=w5261:bool)  [unwired: 1 out]
                n3836 = Absolute Value(x=w5287) -> (abs(x)=w5285:dbl)
                n3837 = case shown="63.." w5279 {
                  tunnel: [2 3 3 1] -> w5272
                  frame 61, 62 {
                  }
                  frame 63.. {
                  }
                  frame ..0 {
                  }
                  frame 10..60, Default {
                  }
                }
                n3838 = case shown="True" w5273 {
                  tunnel: [1 3] -> w5271
                  frame False {
                  }
                  frame True {
                  }
                }
                n3839 = case shown="True" w5276 {
                  tunnel: [1 2] -> w5270
                  frame False {
                  }
                  frame True {
                  }
                }
                n3840 = Multiply(x=1.2 ("y"), y=0.95) -> (x*y=w5249:dbl)
                n3841 = case shown="1..10, Default" w5283 {
                  tunnel: [1 3] -> w5290
                  frame 1..10, Default {
                  }
                  frame 11.. {
                  }
                }
                n3842 = case shown="0..10, Default" w5282 {
                  tunnel: [1 2 3] -> w5289
                  frame 0..10, Default {
                  }
                  frame 11, 12 {
                  }
                  frame 13.. {
                  }
                }
                n3843 = case shown="3601.." w5285 {
                  tunnel: [1 2 3] -> w5284
                  frame 0..3000, Default {
                    # "Normal"
                  }
                  frame 3001..3600 {
                  }
                  frame 3601.. {
                  }
                }
                n3844 = Or(x=w5262, y=w5261) -> (x .or. y?=w5260:bool)
                n3845 = Greater Or Equal?(x=w5265, y=w5249) -> (x >= y?=w5252:bool)
                n3846 = case shown="0, 1, Default" w5265 {
                  tunnel: [1 3] -> w5248
                  frame 0, 1, Default {
                  }
                  frame 2.. {
                  }
                }
                n3847 = case shown="True" w5252 {
                  tunnel: [1 3] -> w5247
                  frame False {
                  }
                  frame True {
                  }
                }
                n3848 = case shown="True" w5260 {
                  tunnel: [1 2] -> w5246
                  frame False {
                  }
                  frame True {
                  }
                }
                n3849 = Build Array(w5272, w5271, w5270) -> (w5269:i32[])
                n3850 = Number To Decimal String(number=w5284) -> (decimal integer string=→"sp_st":string)  [unwired: 1 in]
                n3851 = Array Max & Min(array=w5269) -> (max value=w5266:i32)  [unwired: 3 out]
                "TEMP STATE" <- w5266
                n3852 = Number To Decimal String(number=w5290) -> (decimal integer string=w5293:string)  [unwired: 1 in]
                n3853 = Number To Decimal String(number=w5289) -> (decimal integer string=w5291:string)  [unwired: 1 in]
                n3854 = Number To Decimal String(number=w5266) -> (decimal integer string=→"temp_st":string)  [unwired: 1 in]
                n3855 = Build Array(w5248, w5247, w5246) -> (w5245:i32[])
                n3856 = local write "nl_st"(w5293) -> ()
                n3857 = local write "ff_st"(w5291) -> ()
                n3858 = Number To Decimal String(number=1) -> (decimal integer string=w5288:string)  [unwired: 1 in]
                n3859 = Array Max & Min(array=w5245) -> (max value=w5244:i32)  [unwired: 3 out]
                n3860 = local write "Air temp"(w5288) -> ()
                n3861 = Number To Decimal String(number=w5244) -> (decimal integer string=w5243:string)  [unwired: 1 in]
                n3862 = local write "Stroke Ln 2"(w5243) -> ()
              }
            }
            n3863 = local read "Stroke Ln 2"() -> (w5155:string)
            n3864 = local read "nl_st"() -> (w5161:string)
            n3865 = local read "ff_st"() -> (w5158:string)
            n3866 = local read "sp_st"() -> (w5159:string)
            n3867 = local read "temp_st"() -> (w5160:string)
            n3868 = local read "Air temp"() -> (w5154:string)
            n3869 = Replace Array Subset(array="in", new element #1=w5161, index #1=1 ("index"), new element #2=w5158, index #2=2 ("index"), new element #3=w5160, index #3=3 ("index"), new element #4=w5159, index #4=4 ("index"), new element #5=w5155, index #5=5 ("index"), new element #6=w5154, index #6=6 ("index"), new element #7="Sensor State" ("new element/subarray"), index #7=0 ("index")) -> (→"out":string[])
          }
        }
        n3870 = Wait (ms)(milliseconds to wait=u32 10) -> ()  [unwired: 1 out]
        n3871 = local read "Quit"() -> (w5149:bool)
      }
      n3872 = while {
        stop <- w5124 stop-if-true
        n3873 = local read "run replace"() -> (w5126:bool)
        n3874 = Wait (ms)(milliseconds to wait=u32 100) -> ()  [unwired: 1 out]
        n3875 = Equal?(x="FLAG 2", y=0.0) -> (x = y?=w5127:bool)
        n3876 = case shown="True" w5127 {
          frame False {
          }
          frame True {
            n3877 = local write "FLAG 2"(100.0 ("FLAG 2")) -> ()
            n3878 = call <vilib>:"Read Characters From File.vi"("file path (dialog if empty)"=path "C:/LAB-IQ-NXT/WO 2449 TT.sig", "convert eol? (no:F)"=FALSE ("append to file? (new file:F)")) -> ("character string"=w5130:string)  [unwired: 4 in, 3 out]
            n3879 = call <vilib>:"Read Characters From File.vi"("file path (dialog if empty)"=path "C:/LAB-IQ-NXT/WO 2449 TRH.sig", "convert eol? (no:F)"=FALSE ("append to file? (new file:F)")) -> ("character string"=w5131:string)  [unwired: 4 in, 3 out]
            n3880 = Decimal String To Number(string=w5130) -> (number=w5132:i32)  [unwired: 2 in, 1 out]
            n3881 = local write "Total No. of Tests"(w5132) -> ()
            n3882 = Decimal String To Number(string=w5131) -> (number=w5135:i32)  [unwired: 2 in, 1 out]
            n3883 = local write "SEN.RUN HRS"(w5135) -> ()
          }
        }
        n3884 = case shown="True" w5126 {
          frame False {
          }
          frame True {
            n3885 = Equal?(x="FLAG 4", y=0.0) -> (x = y?=w5139:bool)
            n3886 = case shown="False" w5139 {
              frame False {
                n3887 = Get Date/Time In Seconds() -> (seconds since 1Jan1904=w5145:timestamp)
                n3888 = local read "START 3"() -> (w5143:dbl)
                n3889 = To Double Precision Float(number=w5145) -> (double precision float=w5144:dbl)
                n3890 = Subtract(x=w5144, y=w5143) -> (x-y=→"SENSOR TIME":dbl)
              }
              frame True {
                n3891 = Get Date/Time In Seconds() -> (seconds since 1Jan1904=w5147:timestamp)
                n3892 = local write "FLAG 4"(100.0 ("FLAG")) -> ()
                n3893 = To Double Precision Float(number=w5147) -> (double precision float=→"START 3":dbl)
              }
            }
          }
        }
        n3894 = local read "Quit"() -> (w5124:bool)
      }
      n3895 = while {
        shift-right: [w4924] -> _
        shift-left: _ -> [w4925]
        tunnel: [w4920] -> _
        i -> [w4920]
        stop <- w4919 stop-if-true
        n3896 = Wait (ms)(milliseconds to wait=u32 50 ("Refresh Rate (ms)")) -> ()  [unwired: 1 out]
        n3897 = local read "Json End Flg"() -> (w4921:bool)
        n3898 = Not(x="Upld AR 2") -> ()  [unwired: 1 out]
        n3899 = local read "Upld AR 2"() -> (w4922:bool)
        n3900 = call "Elapsed Time9"("Time Target (s)"="Sen.Upload Rate (s)", "Reset"=FALSE, "Auto Reset"=TRUE) -> ("Time has Elapsed"=w4931:bool)  [unwired: 9 in, 7 out]
        n3901 = Or(x=w4931, y=w4921) -> (x .or. y?=w4927:bool)
        n3902 = case shown="True" w4927 {
          frame False {
          }
          frame True {
            w5023 = "\"SensorName\":\"" ("string")
            w4993 = " \"},{"
            w5018 = "\",\"SensorState\":\""
            w5020 = "\",\"SensorModelNumber\":\"" ("string")
            w5019 = "\",\"SensorRuntimeHours\":\"" ("string")
            n3903 = local read "model num"() -> (w5017:string[])
            n3904 = local read "Sensor name"() -> (w5036:string[])
            n3905 = local read "run"() -> (w5007:string[])
            n3906 = local read "SENSOR TIME"() -> (w4963:dbl)
            n3907 = local read "out"() -> (w4956:string[])
            n3908 = local read "Total No. of Tests"() -> (w4961:dbl)
            n3909 = Select(t=60.0, s="Run test 3", f=3600.0) -> (s? t:f=w4971:dbl)
            n3910 = Index Array(array=w5017, index #1=1 ("index")) -> (element #1=w5016:string, element #2=w5015:string, element #3=w5014:string, element #4=w5013:string, element #5=w5012:string, element #6=w5011:string)  [unwired: 5 in]
            n3911 = Index Array(array=w5007, index #1=1 ("index")) -> (element #1=w5006:string, element #2=w5005:string, element #3=w5004:string, element #4=w5003:string, element #5=w5002:string, element #6=w5001:string)  [unwired: 5 in]
            n3912 = Index Array(array=w5036, index #1=1 ("index")) -> (element #1=w5035:string, element #2=w5034:string, element #3=w5033:string, element #4=w5032:string, element #5=w5022:string, element #6=w5021:string)  [unwired: 5 in]
            n3913 = Index Array(array=w4956, index #1=1 ("index")) -> (element #1=w4988:string, element #2=w4987:string, element #3=w4986:string, element #4=w4985:string, element #5=w4984:string, element #6=w4983:string)  [unwired: 5 in]
            n3914 = local read "SEN.RUN HRS"() -> (w4959:dbl)
            n3915 = Divide(x=w4963, y=w4971) -> (x/y=w4970:dbl)
            n3916 = Increment(x=w4970) -> (x+1=w4966:dbl)
            n3917 = Number To Decimal String(number=w4966) -> (decimal integer string=→"run hrs":string)  [unwired: 1 in]
            n3918 = Divide(x=w4959, y=3600.0 ("f")) -> (x/y=w4954:dbl)
            n3919 = Round To Nearest(number=w4954) -> (nearest integer value=w4952:dbl)
            n3920 = Number To Decimal String(number=w4952) -> (decimal integer string=w4953:string)  [unwired: 1 in]
            n3921 = Number To Decimal String(number=w4961) -> (decimal integer string=w4962:string)  [unwired: 1 in]
            n3922 = local read "Model No"() -> (w4967:string)
            n3923 = local read "UUID"() -> (w5062:string)
            n3924 = local read "Serial No"() -> (w5066:string)
            n3925 = local read "Secret Key"() -> (w5067:string)
            n3926 = Concatenate Strings("\",\"MachineSerialNumber\":\"" ("string"), w5066) -> (w5070:string)
